vi "dfd_Render Complex Root.vi"(0 "display format":T1 items=["Separated Roots", "Combined Roots"], 4 "alignment(left, top)":T2, 5 "format string":string="%.0f", 6 "bracket":cluster{"left":string, "right":string}={"left"="(", "right"=")"}, 7 "Fonts Input":T3(array[cluster]), 8 "variable":string="z", 9 "origin":cluster{"x":i16, "y":i16}, 10 "complex numbers":cdb[](array[numeric]) format="%_2g", 11 "picture in":picture) -> (2 "text rect":T4, 3 "picture out":picture)   [LabVIEW 2017, in "NI_DigFilter_Process.lvlib"]
uses:
  <vilib>/addons/Digital Filter Design/NI_DigFilter_Process.lvlib
  <vilib>/addons/Digital Filter Design/Render.llb/dfd_ZPK Display Format.ctl
  <vilib>/Analysis/polynomials.llb/Unique Numbers and Multiplicity (CDB).vi
  <vilib>/Analysis/NI_AALPro.lvlib
panel:
  in  "Fonts Defaut":T3(array[cluster])=[{"Font Name:"="Tahoma", "Size"=13, "Strikeout?"=FALSE, "Italic?"=FALSE, "Underline?"=FALSE, "Outline?"=FALSE, "Shadow?"=FALSE, "Bold?"=FALSE}, {"Font Name:"="Tahoma", "Size"=13, "Strikeout?"=FALSE, "Italic?"=FALSE, "Underline?"=FALSE, "Outline?"=FALSE, "Shadow?"=FALSE, "Bold?"=FALSE}, {"Font Name:"="Tahoma", "Size"=11, "Strikeout?"=FALSE, "Italic?"=FALSE, "Underline?"=FALSE, "Outline?"=FALSE, "Shadow?"=FALSE, "Bold?"=FALSE}]
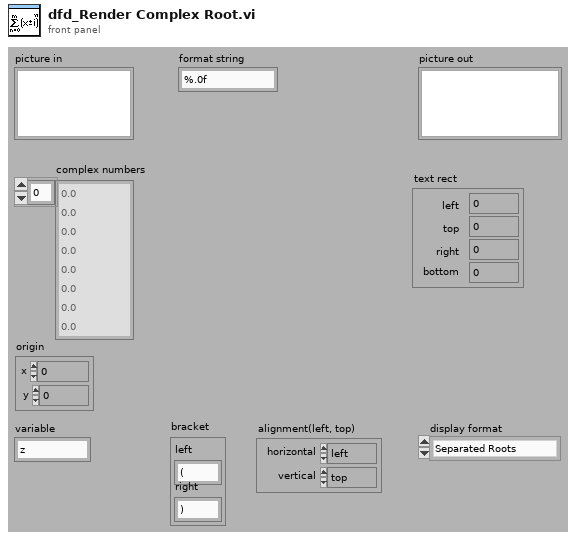
[diagram p1: front panel]
types:
  T1 = typedef "dfd_ZPK Display Format.ctl" = u16
  T2 = cluster{"horizontal":enum16{"left", "center", "right"}, "vertical":enum16{"top", "center", "bottom"}}
  T3 = cluster{"Font Name:":string, "Size":i16, "Strikeout?":bool, "Italic?":bool, "Underline?":bool, "Outline?":bool, "Shadow?":bool, "Bold?":bool}[]
  T4 = cluster{"left":i16, "top":i16, "right":i16, "bottom":i16}
  T5 = enum16{"User-specified Font", "Application Font", "System Font", "Dialog Font"}
  T6 = cluster{"Font Name:":string, "Size":i16, "Strikeout?":bool, "Italic?":bool, "Underline?":bool, "Outline?":bool, "Shadow?":bool, "Bold?":bool}
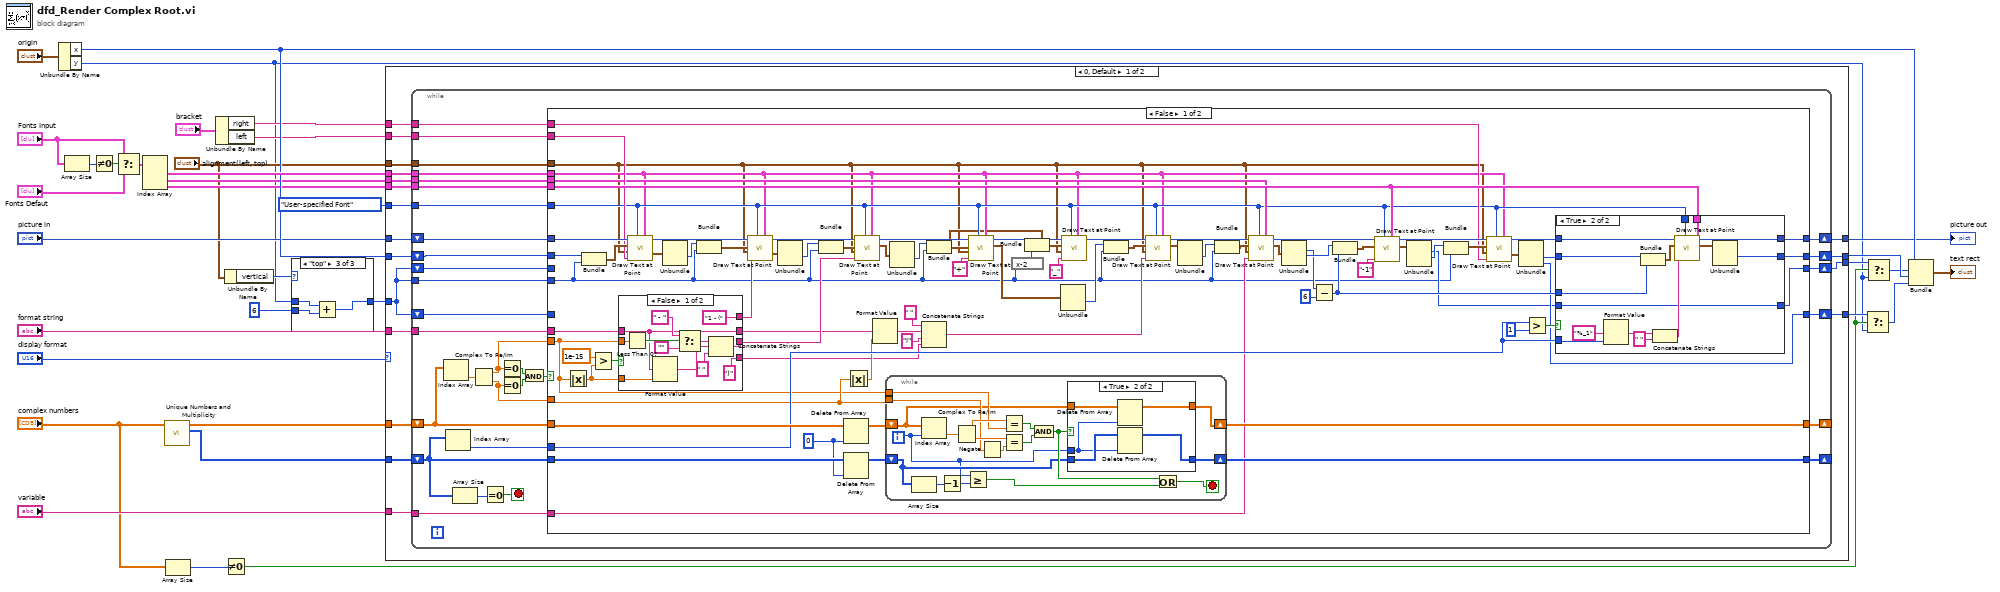
[diagram p0: block diagram]
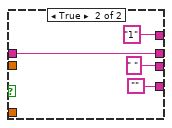
[diagram p2: hidden frame]
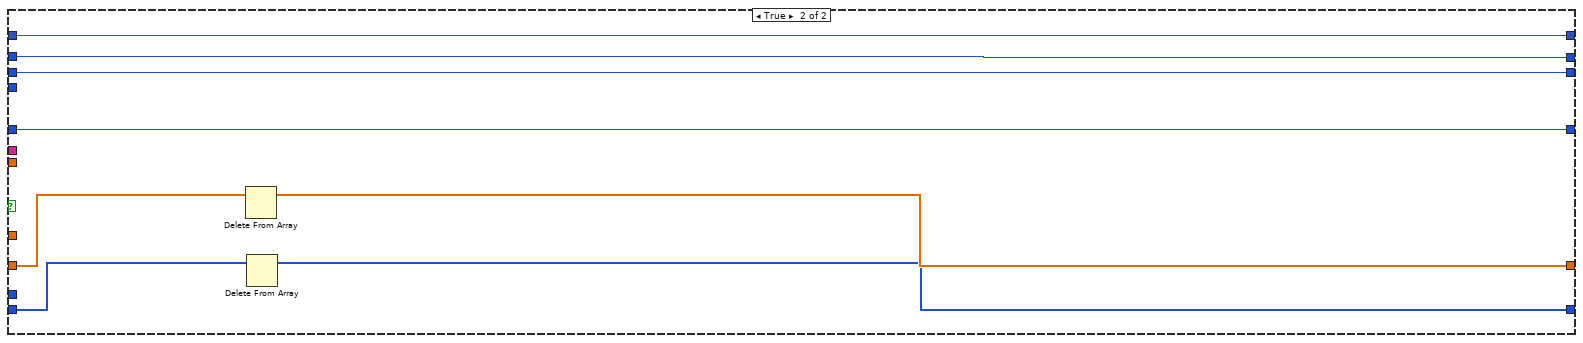
[diagram p5: hidden frame]
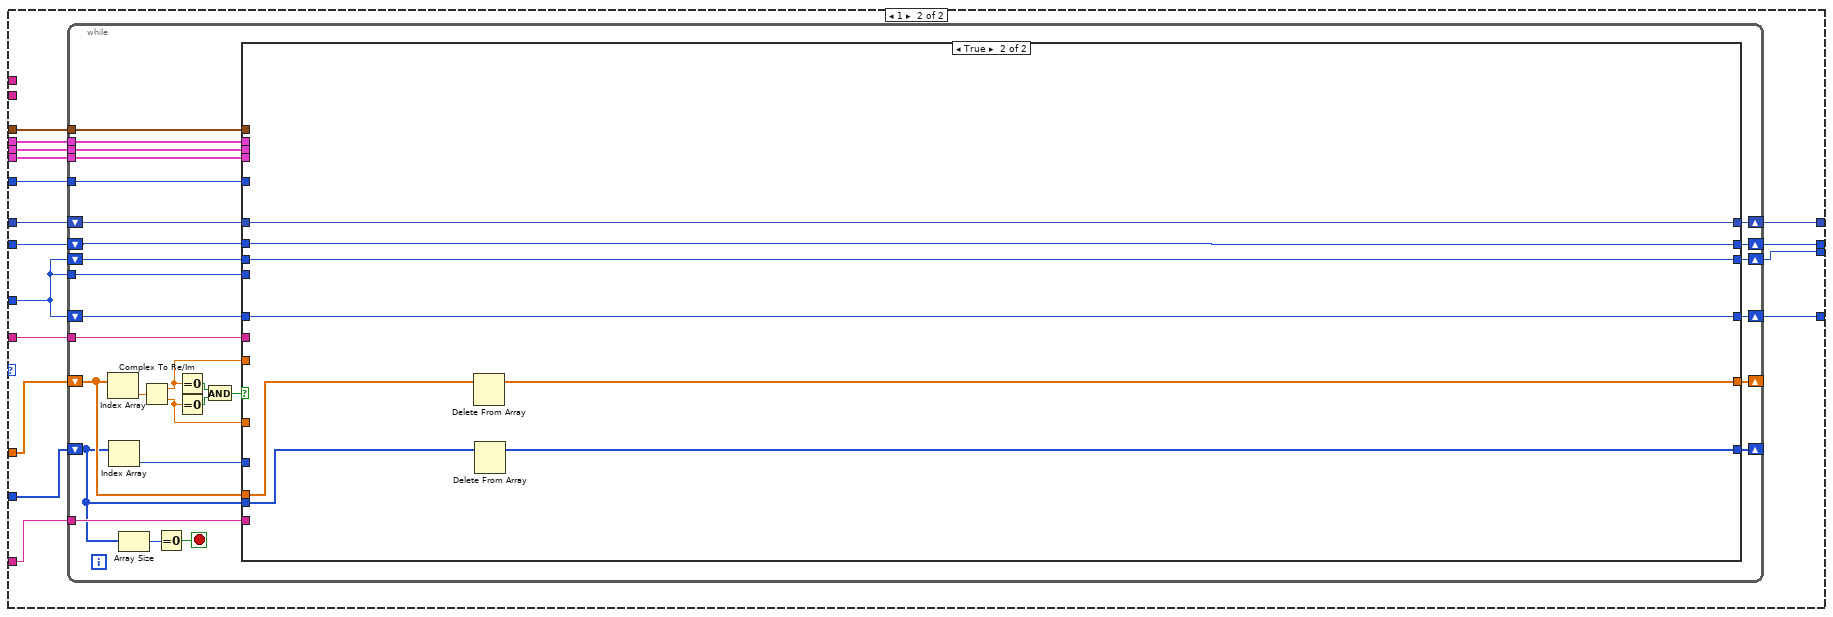
[diagram p6: hidden frame]
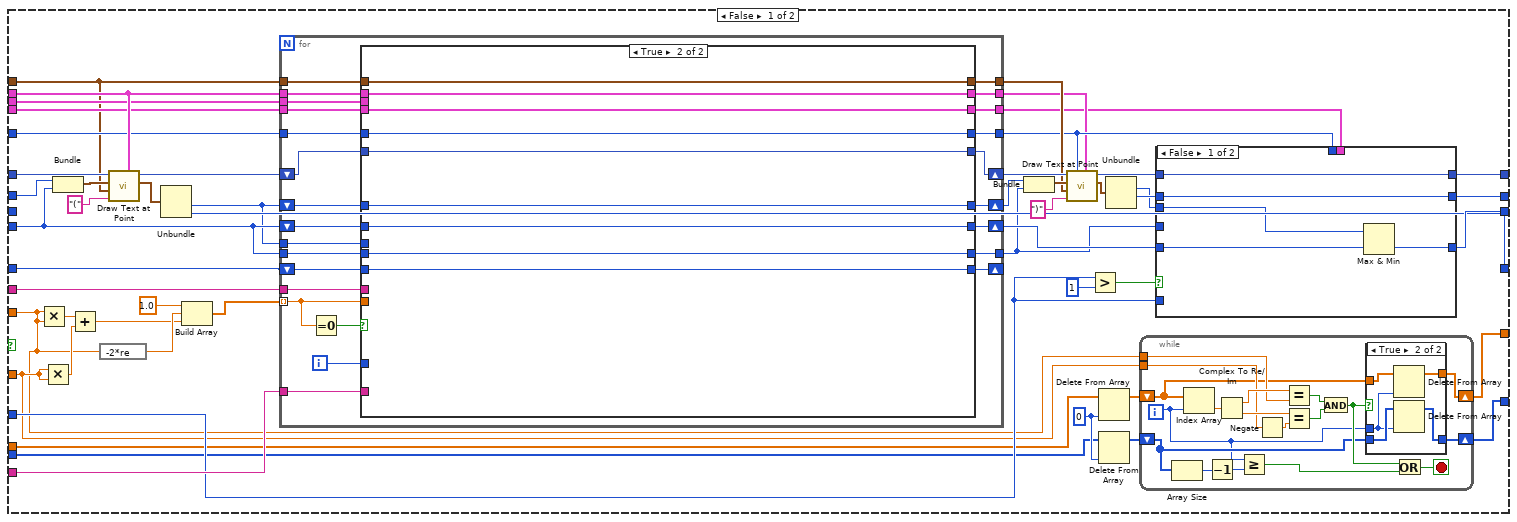
[diagram p7: hidden frame]
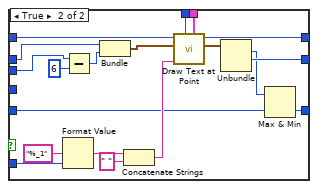
[diagram p9: hidden frame]
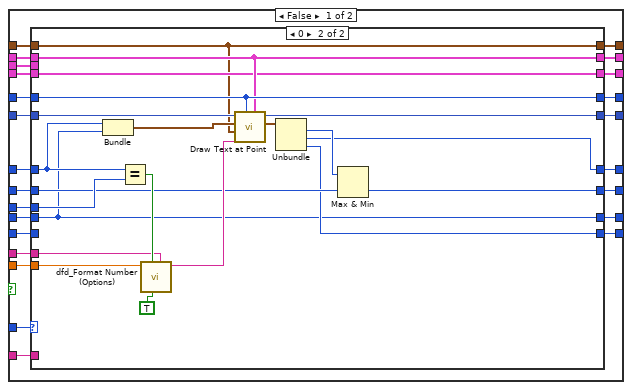
[diagram p10: hidden frame]
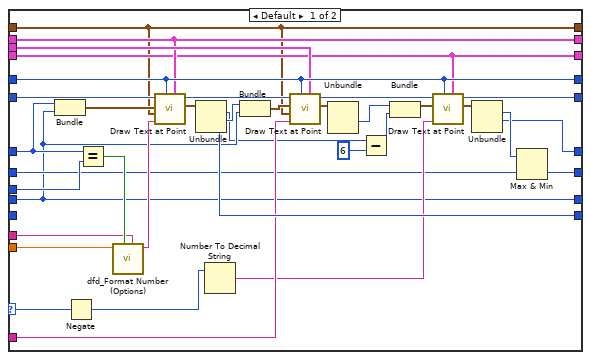
[diagram p11: hidden frame]
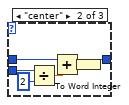
[diagram p13: hidden frame]
diagram:
  n1 = Unbundle By Name("origin") -> ("x"=w26:i16, "y"=w1:i16)
  n2 = Array Size(array="Fonts Input") -> (size(s)=w34:i32)
  n3 = Not Equal To 0?(x=w34) -> (x != 0?=w35:bool)
  n4 = Select(t="Fonts Input", s=w35, f="Fonts Defaut") -> (s? t:f=w32:T3)
  n5 = Index Array(array=w32) -> (element #1=w27:T6, element #2=w20:T6, element #3=w19:T6)  [unwired: 3 in]
  n6 = call-poly <vilib>:"Unique Numbers and Multiplicity.vi"("Complex Numbers"="complex numbers") -> ("Multiplicity"=w18:u32[], "Unique Complex Numbers"=w17:cdb[])  [unwired: 9 out]
  n7 = Array Size(array="complex numbers") -> (size(s)=w7:i32)
  n8 = Unbundle By Name("bracket") -> ("right"=w11:string, "left"=w10:string)
  n9 = Not Equal To 0?(x=w7) -> (x != 0?=w2:bool)
  n10 = Unbundle By Name("alignment(left, top)") -> ("vertical"=w14:enum16{"top", "center", "bottom"})
  n11 = case shown="\"top\"" w14 {
    tunnel: [w36 w37 w44] -> w16
    tunnel: w1 -> [w36 w42 w45]
    tunnel: i16 6 -> [_ w40 w43]
    frame "bottom", Default {
    }
    frame "center" {
      n12 = Divide(x=w40, y=i16 2) -> (x/y=w38:dbl)
      n13 = Add(x=w42, y=w38) -> (x+y=w41:dbl)
      n14 = To Word Integer(number=w41) -> (16bit integer=w37:i16)
    }
    frame "top" {
      n15 = Add(x=w45, y=w43) -> (x+y=w44:i16)
    }
  }
  n16 = case shown="0, Default" "display format" {
    tunnel: "variable" -> [w63 w245]
    tunnel: w27 -> [w62 w254]
    tunnel: w26 -> [w61 w249]
    tunnel: "picture in" -> [w60 w250]
    tunnel: "format string" -> [w59 w247]
    tunnel: T5."User-specified Font" ("desired font(Application)") -> [w58 w251]
    tunnel: [w57 w259] -> w22
    tunnel: [w56 w256] -> w3
    tunnel: [w55 w257] -> w4
    tunnel: [w54 w258] -> w21
    tunnel: w20 -> [w53 w253]
    tunnel: w19 -> [w52 w252]
    tunnel: w18 -> [w51 w244]
    tunnel: w17 -> [w50 w246]
    tunnel: w16 -> [w49 w248]
    tunnel: "alignment(left, top)" -> [w48 w255]
    tunnel: w11 -> [w47 _]
    tunnel: w10 -> [w46 _]
    frame 0, Default {
      n17 = while {
        shift-right: [w79] -> _
        shift-left: w50 -> [w80]
        shift-right: [w78] -> _
        shift-left: w51 -> [w75]
        tunnel: w63 -> [w94]
        tunnel: w49 -> [w93]
        shift-right: [w89] -> w54
        shift-left: w61 -> [w86]
        shift-right: [w88] -> w57
        shift-left: w60 -> [w87]
        tunnel: w62 -> [w85]
        tunnel: w58 -> [w84]
        tunnel: w48 -> [w83]
        tunnel: w59 -> [w82]
        shift-right: [w92] -> w56
        shift-left: w49 -> [w81]
        tunnel: w53 -> [w77]
        tunnel: w52 -> [w76]
        shift-right: [w90] -> w55
        shift-left: w49 -> [w91]
        tunnel: w46 -> [w65]
        tunnel: w47 -> [w64]
        stop <- w73 stop-if-true
        n18 = Index Array(array=w80) -> (element=w72:cdb)  [unwired: 1 in]
        n19 = Index Array(array=w75) -> (element=w66:u32)  [unwired: 1 in]
        n20 = Array Size(array=w75) -> (size(s)=w74:i32)
        n21 = Complex To Re/Im(x + iy=w72) -> (x=w68:dbl, y=w67:dbl)
        n22 = Equal To 0?(x=w74) -> (x = 0?=w73:bool)
        n23 = Equal To 0?(x=w68) -> (x = 0?=w71:bool)
        n24 = Equal To 0?(x=w67) -> (x = 0?=w70:bool)
        n25 = And(x=w71, y=w70) -> (x .and. y?=w69:bool)
        n26 = case shown="False" w69 {
          tunnel: w80 -> [w153 w239]
          tunnel: w75 -> [w152 w238]
          tunnel: w68 -> [w110 _]
          tunnel: w67 -> [w140 _]
          tunnel: w66 -> [w143 _]
          tunnel: w94 -> [w124 _]
          tunnel: w93 -> [w96 _]
          tunnel: [w120 w240] -> w92
          tunnel: w91 -> [_ w241]
          tunnel: [w141 w241] -> w90
          tunnel: [w146 w242] -> w89
          tunnel: [w147 w243] -> w88
          tunnel: w87 -> [w161 w243]
          tunnel: w86 -> [w160 w242]
          tunnel: w85 -> [w103 _]
          tunnel: w84 -> [w104 _]
          tunnel: w83 -> [w97 _]
          tunnel: w82 -> [w136 _]
          tunnel: w81 -> [_ w240]
          tunnel: [w149 w237] -> w79
          tunnel: [w148 w236] -> w78
          tunnel: w77 -> [w106 _]
          tunnel: w76 -> [w119 _]
          tunnel: w65 -> [w115 _]
          tunnel: w64 -> [w114 _]
          frame False {
            w145 = 0 ("index")
            n27 = Absolute Value(x=w110) -> (abs(x)=w109:dbl)
            n28 = Bundle("x"=w160, "y"=w96) -> (w174:cluster{"x":i16, "y":i16})  [unwired: 1 out]
            n29 = Greater?(x=1e-15, y=w109) -> (0:w108:bool)
            n30 = case shown="False" w108 {
              tunnel: [w186 " "] -> w138
              tunnel: w110 -> [w183 _]
              tunnel: ["1 - (" ("string") "1"] -> w137
              tunnel: w136 -> [w180 w192]
              tunnel: [w180 w192] -> w135
              tunnel: [")" ("string") ""] -> w125
              tunnel: w109 -> [w177 _]
              frame False {
                n31 = Less Than 0?(x=w183) -> (x < 0?=w187:bool)
                n32 = Format Value(format string=w180, value (0)=w177) -> (output string=w182:string)  [unwired: 1 out]
                n33 = Select(t=" - " ("string"), s=w187, f="") -> (s? t:f=w185:string)
                n34 = Concatenate Strings(w185, w182, " " ("string")) -> (w186:string)
              }
              frame True {
              }
            }
            n35 = call <vilib>:"Draw Text at Point.vi"("[user-specified font]"=w103, "desired font(Application)"=w104, "text"=w115, "alignment(left, top)"=w97, "origin"=w174, "picture"=w161) -> ("text rect"=w169:T4, "new picture"=w168:picture)  [unwired: 3 in, 1 out]
            n36 = Unbundle(w169) -> ("right"=w172:i16)  [unwired: 3 out]
            n37 = Bundle("right"=w172, "y"=w96) -> (w170:cluster{"right":i16, "y":i16})  [unwired: 1 out]
            n38 = call <vilib>:"Draw Text at Point.vi"("[user-specified font]"=w103, "desired font(Application)"=w104, "text"=w137, "alignment(left, top)"=w97, "origin"=w170, "picture"=w168) -> ("text rect"=w171:T4, "new picture"=w176:picture)  [unwired: 3 in, 1 out]
            n39 = Unbundle(w171) -> ("right"=w173:i16)  [unwired: 3 out]
            n40 = Bundle("right"=w173, "y"=w96) -> (w175:cluster{"right":i16, "y":i16})  [unwired: 1 out]
            n41 = Delete From Array(array=w153, index=w145) -> (array with subset deleted=w151:cdb[])  [unwired: 1 in, 1 out]
            n42 = Delete From Array(array=w152, index=w145) -> (array with subset deleted=w150:u32[])  [unwired: 1 in, 1 out]
            n43 = Absolute Value(x=w140) -> (abs(x)=w139:dbl)
            n44 = call <vilib>:"Draw Text at Point.vi"("[user-specified font]"=w103, "desired font(Application)"=w104, "text"=w138, "alignment(left, top)"=w97, "origin"=w175, "picture"=w176) -> ("text rect"=w167:T4, "new picture"=w165:picture)  [unwired: 3 in, 1 out]
            n45 = Format Value(format string=w135, value (0)=w139) -> (output string=w159:string)  [unwired: 1 out]
            n46 = while {
              tunnel: w140 -> [w223]
              tunnel: w110 -> [w226]
              shift-right: [w218] -> w149
              shift-left: w151 -> [w219]
              shift-right: [w217] -> w148
              shift-left: w150 -> [w216]
              i -> [w213]
              stop <- w211 stop-if-true
              n47 = Array Size(array=w216) -> (size(s)=w214:i32)
              n48 = Index Array(array=w219, index=w213) -> (element=w228:cdb)
              n49 = Decrement(x=w214) -> (x-1=w215:i32)
              n50 = Complex To Re/Im(x + iy=w228) -> (x=w227:dbl, y=w225:dbl)
              n51 = Greater Or Equal?(x=w213, y=w215) -> (x >= y?=w212:bool)
              n52 = Negate(x=w223) -> (-x=w224:dbl)
              n53 = Equal?(x=w227, y=w226) -> (x = y?=w222:bool)
              n54 = Equal?(x=w225, y=w224) -> (x = y?=w221:bool)
              n55 = And(x=w222, y=w221) -> (x .and. y?=w220:bool)
              n56 = case shown="True" w220 {
                tunnel: w216 -> [w229 w234]
                tunnel: w219 -> [w230 w235]
                tunnel: w213 -> [_ w233]
                tunnel: [w230 w232] -> w218
                tunnel: [w229 w231] -> w217
                frame False {
                }
                frame True {
                  n57 = Delete From Array(array=w235, index=w233) -> (array with subset deleted=w232:cdb[])  [unwired: 1 in, 1 out]
                  n58 = Delete From Array(array=w234, index=w233) -> (array with subset deleted=w231:u32[])  [unwired: 1 in, 1 out]
                }
              }
              n59 = Or(x=w220, y=w212) -> (x .or. y?=w211:bool)
            }
            n60 = Unbundle(w167) -> ("right"=w112:i16)  [unwired: 3 out]
            n61 = Concatenate Strings(" ", w159, "i" ("string"), w125) -> (w157:string)
            n62 = Bundle("right"=w112, "y"=w96) -> (w98:cluster{"right":i16, "y":i16})  [unwired: 1 out]
            n63 = call <vilib>:"Draw Text at Point.vi"("[user-specified font]"=w103, "desired font(Application)"=w104, "text"="+", "alignment(left, top)"=w97, "origin"=w98, "picture"=w165) -> ("text rect"=w166:T4, "new picture"=w105:picture)  [unwired: 3 in, 1 out]
            n64 = expression code="x-2"(w96) -> (w95:i16)
            n65 = Bundle(cluster=w98, "y"=w95) -> (w99:cluster{"right":i16, "y":i16})  [unwired: 1 out]
            n66 = Unbundle(w166) -> ("right"=w164:i16)  [unwired: 3 out]
            n67 = call <vilib>:"Draw Text at Point.vi"("[user-specified font]"=w103, "desired font(Application)"=w104, "text"="_", "alignment(left, top)"=w97, "origin"=w99, "picture"=w105) -> ("new picture"=w102:picture)  [unwired: 3 in, 2 out]
            n68 = Bundle("right"=w164, "y"=w96) -> (w162:cluster{"right":i16, "y":i16})  [unwired: 1 out]
            n69 = call <vilib>:"Draw Text at Point.vi"("[user-specified font]"=w103, "desired font(Application)"=w104, "text"=w157, "alignment(left, top)"=w97, "origin"=w162, "picture"=w102) -> ("text rect"=w163:T4, "new picture"=w154:picture)  [unwired: 3 in, 1 out]
            n70 = Unbundle(w163) -> ("right"=w156:i16)  [unwired: 3 out]
            n71 = Bundle("right"=w156, "y"=w96) -> (w155:cluster{"right":i16, "y":i16})  [unwired: 1 out]
            n72 = call <vilib>:"Draw Text at Point.vi"("[user-specified font]"=w106, "desired font(Application)"=w104, "text"=w124, "alignment(left, top)"=w97, "origin"=w155, "picture"=w154) -> ("text rect"=w118:T4, "new picture"=w128:picture)  [unwired: 3 in, 1 out]
            n73 = Unbundle(w118) -> ("top"=w113:i16, "right"=w117:i16)  [unwired: 2 out]
            n74 = Subtract(x=w113, y=i16 6) -> (x-y=w121:i16)
            n75 = Bundle("right"=w117, w121) -> (w133:cluster{"right":i16, i16})  [unwired: 1 out]
            n76 = call <vilib>:"Draw Text at Point.vi"("[user-specified font]"=w119, "desired font(Application)"=w104, "text"="-1", "origin"=w133, "picture"=w128) -> ("text rect"=w134:T4, "new picture"=w130:picture)  [unwired: 4 in, 1 out]
            n77 = Unbundle(w134) -> ("top"=w116:i16, "right"=w132:i16)  [unwired: 2 out]
            n78 = Bundle("right"=w132, "y"=w96) -> (w131:cluster{"right":i16, "y":i16})  [unwired: 1 out]
            n79 = call <vilib>:"Draw Text at Point.vi"("[user-specified font]"=w103, "desired font(Application)"=w104, "text"=w114, "alignment(left, top)"=w97, "origin"=w131, "picture"=w130) -> ("text rect"=w129:T4, "new picture"=w126:picture)  [unwired: 3 in, 1 out]
            n80 = Unbundle(w129) -> ("right"=w127:i16, "bottom"=w120:i16)  [unwired: 2 out]
            n81 = Greater?(x=w143, y=u32 1) -> (0:w144:bool)
            n82 = case shown="True" w144 {
              tunnel: w127 -> [w194 w209]
              tunnel: w119 -> [_ w208]
              tunnel: w126 -> [w195 w207]
              tunnel: w143 -> [_ w205]
              tunnel: [w195 w204] -> w147
              tunnel: [w194 w203] -> w146
              tunnel: [w193 w196] -> w141
              tunnel: w121 -> [_ w198]
              tunnel: w104 -> [_ w197]
              tunnel: w116 -> [w193 w196]
              frame False {
              }
              frame True {
                n83 = Format Value(format string="%_1", value (0)=w205) -> (output string=w201:string)  [unwired: 1 out]
                n84 = Bundle("right"=w209, w198) -> (w206:cluster{"right":i16, i16})  [unwired: 1 out]
                n85 = Concatenate Strings(w201, " " ("string")) -> (w199:string)
                n86 = call <vilib>:"Draw Text at Point.vi"("[user-specified font]"=w208, "desired font(Application)"=w197, "text"=w199, "origin"=w206, "picture"=w207) -> ("text rect"=w210:T4, "new picture"=w204:picture)  [unwired: 4 in, 1 out]
                n87 = Unbundle(w210) -> ("right"=w203:i16)  [unwired: 3 out]
              }
            }
          }
          frame True {
            n88 = Delete From Array(array=w239) -> (array with subset deleted=w237:cdb[])  [unwired: 2 in, 1 out]
            n89 = Delete From Array(array=w238) -> (array with subset deleted=w236:u32[])  [unwired: 2 in, 1 out]
          }
        }
      }
    }
    frame 1 {
      n90 = while {
        shift-right: [w275] -> _
        shift-left: w246 -> [w276]
        shift-right: [w274] -> _
        shift-left: w244 -> [w271]
        tunnel: w245 -> [w288]
        tunnel: w248 -> [w287]
        shift-right: [w284] -> w258
        shift-left: w249 -> [w281]
        shift-right: [w283] -> w259
        shift-left: w250 -> [w282]
        tunnel: w254 -> [w280]
        tunnel: w251 -> [w279]
        tunnel: w255 -> [w278]
        tunnel: w247 -> [w277]
        tunnel: w253 -> [w273]
        tunnel: w252 -> [w272]
        shift-right: [w285] -> w257
        shift-left: w248 -> [w286]
        shift-right: [w262] -> w256
        shift-left: w248 -> [w261]
        stop <- w269 stop-if-true
        n91 = Index Array(array=w276) -> (element=w260:cdb)  [unwired: 1 in]
        n92 = Index Array(array=w271) -> (element=w263:u32)  [unwired: 1 in]
        n93 = Array Size(array=w271) -> (size(s)=w270:i32)
        n94 = Complex To Re/Im(x + iy=w260) -> (x=w265:dbl, y=w264:dbl)
        n95 = Equal To 0?(x=w270) -> (x = 0?=w269:bool)
        n96 = Equal To 0?(x=w265) -> (x = 0?=w268:bool)
        n97 = Equal To 0?(x=w264) -> (x = 0?=w267:bool)
        n98 = And(x=w268, y=w267) -> (x .and. y?=w266:bool)
        n99 = case shown="True" w266 {
          tunnel: w276 -> [w309 w509]
          tunnel: w271 -> [w308 w508]
          tunnel: w265 -> [w293 _]
          tunnel: w264 -> [w294 _]
          tunnel: w263 -> [w314 _]
          tunnel: w288 -> [w329 _]
          tunnel: w287 -> [w330 _]
          tunnel: w286 -> [_ w510]
          tunnel: [w312 w510] -> w285
          tunnel: [w313 w511] -> w284
          tunnel: [w321 w512] -> w283
          tunnel: w282 -> [w335 w512]
          tunnel: w281 -> [w337 w511]
          tunnel: w280 -> [w334 _]
          tunnel: w279 -> [w331 _]
          tunnel: w278 -> [w328 _]
          tunnel: w277 -> [w300 _]
          tunnel: [w305 w507] -> w275
          tunnel: [w304 w506] -> w274
          tunnel: w273 -> [w333 _]
          tunnel: w272 -> [w332 _]
          tunnel: [w311 w505] -> w262
          tunnel: w261 -> [w299 w505]
          frame False {
            w310 = 0 ("index")
            n100 = Multiply(x=w293, y=w293) -> (x*y=w296:dbl)
            n101 = Multiply(x=w294, y=w294) -> (x*y=w295:dbl)
            n102 = Bundle("x"=w337, "y"=w330) -> (w338:cluster{"x":i16, "y":i16})  [unwired: 1 out]
            n103 = Add(x=w296, y=w295) -> (x+y=w289:dbl)
            n104 = expression code="-2*re"(w293) -> (w290:dbl)
            n105 = call <vilib>:"Draw Text at Point.vi"("[user-specified font]"=w334, "text"="(", "alignment(left, top)"=w328, "origin"=w338, "picture"=w335) -> ("text rect"=w340:T4, "new picture"=w336:picture)  [unwired: 4 in, 1 out]
            n106 = Unbundle(w340) -> ("right"=w301:i16, "bottom"=w311:i16)  [unwired: 2 out]
            n107 = Build Array(1.0 ("element"), w290, w289) -> (w292:dbl[])
            n108 = for {
              tunnel: w292 -> [w413] mode=indexing
              shift-right: [w401] -> w324
              shift-left: w336 -> [w402]
              shift-right: [w399] -> w323
              shift-left: w301 -> [w412]
              tunnel: w334 -> [w406]
              tunnel: w333 -> [w405]
              tunnel: w332 -> [w404]
              tunnel: w331 -> [w403]
              shift-right: [w397] -> w298
              shift-left: w330 -> [w398]
              tunnel: w301 -> [w411]
              tunnel: w330 -> [w410]
              shift-right: [w409] -> _
              shift-left: w299 -> [w400]
              tunnel: w329 -> [w408]
              tunnel: w328 -> [w407]
              tunnel: [w396] -> w315
              tunnel: [w395] -> w320
              tunnel: [w394] -> w297
              tunnel: [w393] -> w303
              tunnel: [w392] -> w302
              tunnel: w300 -> [w391]
              i -> [w390]
              n109 = Equal To 0?(x=w413) -> (x = 0?=w414:bool)
              n110 = case shown="True" w414 {
                tunnel: w390 -> [w438 _]
                tunnel: w413 -> [w437 _]
                tunnel: w412 -> [w436 w502]
                tunnel: w411 -> [w435 _]
                tunnel: w410 -> [w434 w498]
                tunnel: [w433 w504] -> w409
                tunnel: w408 -> [w432 _]
                tunnel: w407 -> [w431 w499]
                tunnel: w406 -> [w430 w497]
                tunnel: w405 -> [w429 _]
                tunnel: w404 -> [w428 w496]
                tunnel: w403 -> [w427 w500]
                tunnel: w402 -> [w426 w503]
                tunnel: [w425 w503] -> w401
                tunnel: w400 -> [w424 w504]
                tunnel: [w422 w502] -> w399
                tunnel: w398 -> [w423 w501]
                tunnel: [w421 w501] -> w397
                tunnel: [w420 w500] -> w396
                tunnel: [w419 w499] -> w395
                tunnel: [w418 w498] -> w394
                tunnel: [w417 w497] -> w393
                tunnel: [w416 w496] -> w392
                tunnel: w391 -> [w415 _]
                frame False {
                  n111 = case shown="0" w438 {
                    selector: w438 -> [w441 _]
                    tunnel: w437 -> [w460 w490]
                    tunnel: w436 -> [w458 w487]
                    tunnel: w435 -> [w459 w489]
                    tunnel: w434 -> [w447 w479]
                    tunnel: [w457 w481] -> w433
                    tunnel: w432 -> [w456 _]
                    tunnel: w431 -> [w443 w476]
                    tunnel: w430 -> [w445 w478]
                    tunnel: w429 -> [w446 _]
                    tunnel: w428 -> [w444 w477]
                    tunnel: w427 -> [w448 w480]
                    tunnel: w426 -> [w454 w488]
                    tunnel: [w453 w486] -> w425
                    tunnel: w424 -> [_ _]
                    tunnel: w423 -> [w452 w483]
                    tunnel: [w450 w482] -> w422
                    tunnel: [w449 w484] -> w421
                    tunnel: [w448 w480] -> w420
                    tunnel: [w443 w476] -> w419
                    tunnel: [w447 w479] -> w418
                    tunnel: [w445 w478] -> w417
                    tunnel: [w444 w477] -> w416
                    tunnel: w415 -> [w442 w475]
                    frame Default {
                      n112 = Bundle("right"=w458, "y"=w447) -> (w472:cluster{"right":i16, "y":i16})  [unwired: 1 out]
                      n113 = Negate(x=w441) -> (-x=w440:i32)
                      n114 = Equal?(x=w458, y=w459) -> (x = y?=w461:bool)
                      n115 = call <vilib>:"dfd_Format Number (Options).vi"("format string"=w442, "Is Higher Coeffiecient?"=w461, "Coefficient"=w460) -> ("String Coefficient"=w474:string)  [unwired: 1 in, 7 out]
                      n116 = call <vilib>:"Draw Text at Point.vi"("[user-specified font]"=w445, "desired font(Application)"=w448, "text"=w474, "alignment(left, top)"=w443, "origin"=w472, "picture"=w454) -> ("text rect"=w473:T4, "new picture"=w467:picture)  [unwired: 3 in, 1 out]
                      n117 = Unbundle(w473) -> ("top"=w439:i16, "right"=w463:i16, "bottom"=w457:i16)  [unwired: 1 out]
                      n118 = Number To Decimal String(number=w440) -> (decimal integer string=w455:string)  [unwired: 1 out]
                      n119 = Bundle("right"=w463, "y"=w447) -> (w468:cluster{"right":i16, "y":i16})  [unwired: 1 out]
                      n120 = call <vilib>:"Draw Text at Point.vi"("[user-specified font]"=w446, "desired font(Application)"=w448, "text"=w456, "alignment(left, top)"=w443, "origin"=w468, "picture"=w467) -> ("text rect"=w465:T4, "new picture"=w466:picture)  [unwired: 3 in, 1 out]
                      n121 = Unbundle(w465) -> ("right"=w462:i16)  [unwired: 3 out]
                      n122 = Subtract(x=w439, y=i16 6) -> (x-y=w470:i16)
                      n123 = Bundle("right"=w462, w470) -> (w471:cluster{"right":i16, i16})  [unwired: 1 out]
                      n124 = call <vilib>:"Draw Text at Point.vi"("[user-specified font]"=w444, "desired font(Application)"=w448, "text"=w455, "origin"=w471, "picture"=w466) -> ("text rect"=w464:T4, "new picture"=w453:picture)  [unwired: 4 in, 1 out]
                      n125 = Unbundle(w464) -> ("top"=w451:i16, "right"=w450:i16)  [unwired: 2 out]
                      n126 = Max & Min(x=w451, y=w452) -> (min(x,y)=w449:i16)  [unwired: 1 out]
                    }
                    frame 0 {
                      n127 = Bundle("right"=w487, "y"=w479) -> (w494:cluster{"right":i16, "y":i16})  [unwired: 1 out]
                      n128 = Equal?(x=w487, y=w489) -> (x = y?=w493:bool)
                      n129 = call <vilib>:"dfd_Format Number (Options).vi"("format string"=w475, "Is Lower Coefficient?"=TRUE ("Is Lower Coeffiecient? 2"), "Is Higher Coeffiecient?"=w493, "Coefficient"=w490) -> ("String Coefficient"=w492:string)  [unwired: 7 out]
                      n130 = call <vilib>:"Draw Text at Point.vi"("[user-specified font]"=w478, "desired font(Application)"=w480, "text"=w492, "alignment(left, top)"=w476, "origin"=w494, "picture"=w488) -> ("text rect"=w495:T4, "new picture"=w486:picture)  [unwired: 3 in, 1 out]
                      n131 = Unbundle(w495) -> ("top"=w485:i16, "right"=w482:i16, "bottom"=w481:i16)  [unwired: 1 out]
                      n132 = Max & Min(x=w485, y=w483) -> (min(x,y)=w484:i16)  [unwired: 1 out]
                    }
                  }
                }
                frame True {
                }
              }
            }
            n133 = Bundle("right"=w323, "y"=w297) -> (w326:cluster{"right":i16, "y":i16})  [unwired: 1 out]
            n134 = call <vilib>:"Draw Text at Point.vi"("[user-specified font]"=w303, "desired font(Application)"=w315, "text"=")", "alignment(left, top)"=w320, "origin"=w326, "picture"=w324) -> ("text rect"=w325:T4, "new picture"=w322:picture)  [unwired: 3 in, 1 out]
            n135 = Greater?(x=w314, y=u32 1) -> (0:w316:bool)
            n136 = Delete From Array(array=w309, index=w310) -> (array with subset deleted=w307:cdb[])  [unwired: 1 in, 1 out]
            n137 = Delete From Array(array=w308, index=w310) -> (array with subset deleted=w306:u32[])  [unwired: 1 in, 1 out]
            n138 = Unbundle(w325) -> ("top"=w318:i16, "right"=w319:i16)  [unwired: 2 out]
            n139 = while {
              tunnel: w294 -> [w353]
              tunnel: w293 -> [w356]
              shift-right: [w348] -> w305
              shift-left: w307 -> [w349]
              shift-right: [w347] -> w304
              shift-left: w306 -> [w346]
              i -> [w343]
              stop <- w341 stop-if-true
              n140 = Array Size(array=w346) -> (size(s)=w344:i32)
              n141 = Index Array(array=w349, index=w343) -> (element=w358:cdb)
              n142 = Decrement(x=w344) -> (x-1=w345:i32)
              n143 = Complex To Re/Im(x + iy=w358) -> (x=w357:dbl, y=w355:dbl)
              n144 = Greater Or Equal?(x=w343, y=w345) -> (x >= y?=w342:bool)
              n145 = Negate(x=w353) -> (-x=w354:dbl)
              n146 = Equal?(x=w357, y=w356) -> (x = y?=w352:bool)
              n147 = Equal?(x=w355, y=w354) -> (x = y?=w351:bool)
              n148 = And(x=w352, y=w351) -> (x .and. y?=w350:bool)
              n149 = case shown="True" w350 {
                tunnel: w346 -> [w359 w364]
                tunnel: w349 -> [w360 w365]
                tunnel: w343 -> [_ w363]
                tunnel: [w360 w362] -> w348
                tunnel: [w359 w361] -> w347
                frame False {
                }
                frame True {
                  n150 = Delete From Array(array=w365, index=w363) -> (array with subset deleted=w362:cdb[])  [unwired: 1 in, 1 out]
                  n151 = Delete From Array(array=w364, index=w363) -> (array with subset deleted=w361:u32[])  [unwired: 1 in, 1 out]
                }
              }
              n152 = Or(x=w350, y=w342) -> (x .or. y?=w341:bool)
            }
            n153 = case shown="False" w316 {
              tunnel: w319 -> [w369 w388]
              tunnel: w322 -> [w370 w387]
              tunnel: w314 -> [_ w383]
              tunnel: [w370 w382] -> w321
              tunnel: [w369 w381] -> w313
              tunnel: w298 -> [w367 w375]
              tunnel: [w366 w376] -> w312
              tunnel: w318 -> [w368 w371]
              tunnel: w297 -> [_ _]
              tunnel: w315 -> [_ w373]
              tunnel: w302 -> [_ w372]
              frame False {
                n154 = Max & Min(x=w368, y=w367) -> (min(x,y)=w366:i16)  [unwired: 1 out]
              }
              frame True {
                n155 = Format Value(format string="%_1", value (0)=w383) -> (output string=w379:string)  [unwired: 1 out]
                n156 = Subtract(x=w371, y=i16 6) -> (x-y=w385:i16)
                n157 = Bundle("right"=w388, w385) -> (w384:cluster{"right":i16, i16})  [unwired: 1 out]
                n158 = Concatenate Strings(w379, " " ("string")) -> (w377:string)
                n159 = call <vilib>:"Draw Text at Point.vi"("[user-specified font]"=w372, "desired font(Application)"=w373, "text"=w377, "origin"=w384, "picture"=w387) -> ("text rect"=w389:T4, "new picture"=w382:picture)  [unwired: 4 in, 1 out]
                n160 = Unbundle(w389) -> ("top"=w374:i16, "right"=w381:i16)  [unwired: 2 out]
                n161 = Max & Min(x=w374, y=w375) -> (min(x,y)=w376:i16)  [unwired: 1 out]
              }
            }
          }
          frame True {
            n162 = Delete From Array(array=w509) -> (array with subset deleted=w507:cdb[])  [unwired: 2 in, 1 out]
            n163 = Delete From Array(array=w508) -> (array with subset deleted=w506:u32[])  [unwired: 2 in, 1 out]
          }
        }
      }
    }
  }
  "picture out" <- w22
  n164 = Select(t=w3, s=w2, f=w1) -> (s? t:f=w6:i16)
  n165 = Select(t=w4, s=w2, f=w1) -> (s? t:f=w5:i16)
  n166 = Bundle("x"=w26, "y"=w5, "x"=w21, "y"=w6) -> (→"text rect":cluster{"x":i16, "y":i16, "x":i16, "y":i16})  [unwired: 1 out]
